vi "Acquire Data.vi"(8 "error in (no error)":errorcluster, 11 "DAQmx Force Sensor in":refnum<class "DAQmx Force Sensor.lvclass">) -> (0 "error out":errorcluster, 3 "DAQmx Force Sensor out":refnum<class "DAQmx Force Sensor.lvclass">)   [LabVIEW 2020, in "DAQmx Force Sensor.lvclass"]
uses:
  DAQmx Force Sensor.lvclass
  C:/Users/jharw/Documents/1 Folder to Rule them All/UMD/Inflation-Apparatus/src/Hardware/Sensors/Force Sensors/Force Sensor.lvclass
  DAQmx Force Sensor.lvclass/DAQmx Force Sensor.ctl
  Force Sensor.lvclass/Force Sensor.ctl
  <vilib>/DAQmx/read.llb/DAQmx Read (Analog 1D DBL 1Chan NSamp).vi
  <vilib>/DAQmx/miscellaneous.llb/DAQmx Fill In Error Info.vi
  Force Sensor.lvclass
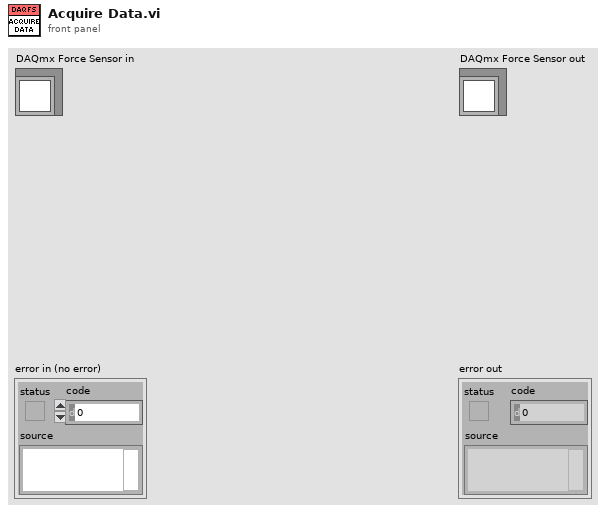
[diagram p1: front panel]
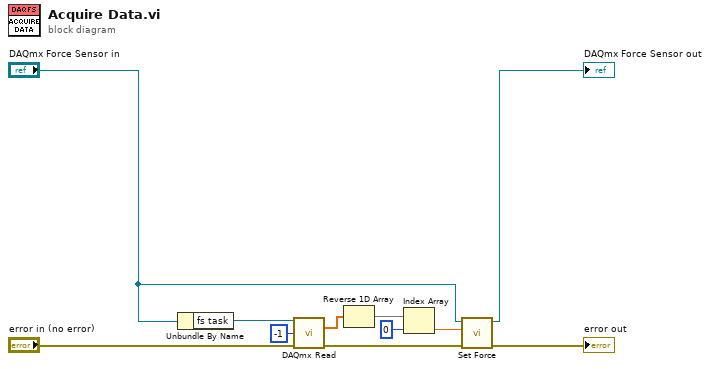
[diagram p0: block diagram]
diagram:
  n1 = Unbundle By Name("DAQmx Force Sensor in") -> ("fs task"=w7:refnum<k21>)
  n2 = call-poly <vilib>:"DAQmx Read.vi"("task/channels in"=w7, "number of samples per channel"=-1, "error in"="error in (no error)") -> ("data"=w11:dbl[], "error out"=w4:errorcluster)  [unwired: 10 in, 1 out]
  n3 = Reverse 1D Array(array=w11) -> (reversed array=w10:dbl[])
  n4 = Index Array ("Take most recent data point")(array=w10, index=0) -> (element=w5:dbl)
  n5 = call "Set Force.vi"("error in (no error)"=w4, "force (V)"=w5, "Force Sensor in"="DAQmx Force Sensor in") -> ("error out"=→"error out":errorcluster, "Force Sensor out"=→"DAQmx Force Sensor out":refnum<class "DAQmx Force Sensor.lvclass">)  [unwired: 7 in]
